vi "Generate Method Description.vi"(8 "error in (no error)":errorcluster, 10 "Test Method Result In":T1, 11 "Test Tree In":refnum<class "Test Result Tree.lvclass">) -> (0 "error out":errorcluster, 3 "Test Tree Out":refnum<class "Test Result Tree.lvclass">)   [LabVIEW 2020, in "Test Result Tree.lvclass"]
uses:
  Test Result Tree/Test Result Tree.lvclass
  Result Types/Method Result/Method Result.ctl
  Rewrite Project/Result/Status.ctl
  Result Types/Assertion Result/Assertion Result.ctl
  Result Types/Assertion Result/Public/TypeDefs/Assertion Type.ctl
  C:/Git/astemes-lunit/source/Framework/Helper Classes/Test Tree/Test Tree.lvclass
  Test Tree.lvclass/Test Tree.ctl
  Test Tree.lvclass
  Result Types/Assertion Result/Assertion Result.lvlib
  Result Types/Method Result/Method Result.lvlib
  Rewrite Project/Result/Result.lvlib
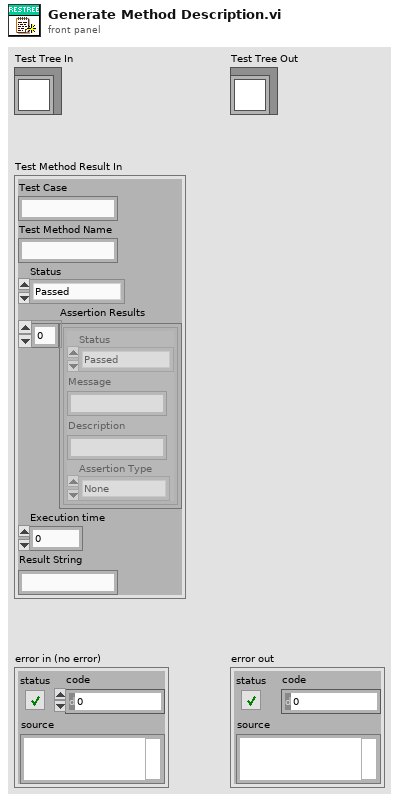
[diagram p1: front panel]
types:
  T1 = typedef "Method Result.lvlib/Method Result.ctl" = cluster{"Test Case":string, "Test Method Name":string, "Status":T2, "Assertion Results":T3[], "Execution time":dbl, "Result String":string}
  T2 = typedef "Result.lvlib/Status.ctl" = enum16{"Passed", "Failed", "Error", "Skipped", "Setup Error", "Broken", "Teardown Error"}
  T3 = typedef "Assertion Result.lvlib/Assertion Result.ctl" = cluster{"Status":T2, "Message":string, "Description":string, "Assertion Type":T4}
  T4 = typedef "Result.lvlib/Assertion Type.ctl" = enum16{"None", "Pass", "Fail", "Skip", "Pass if Equal", "Fail if Equal", "Pass if Error", "Fail if Error", "Pass if", "Fail if"}
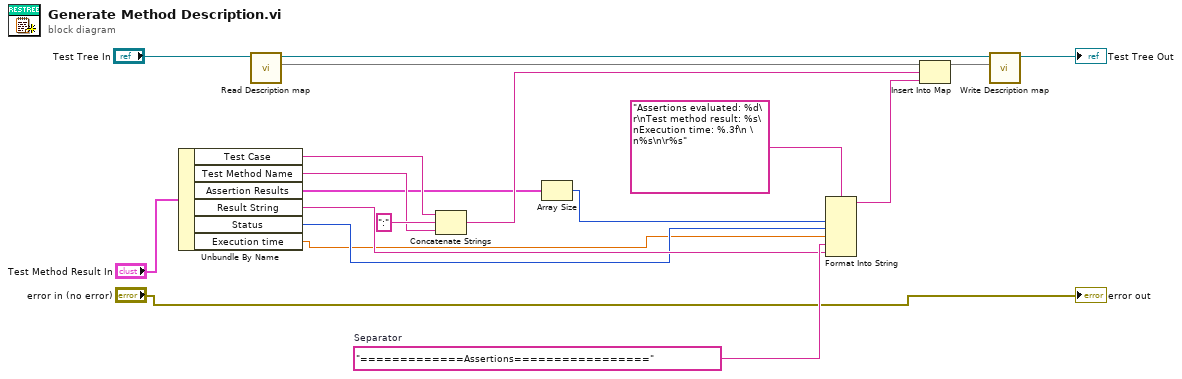
[diagram p0: block diagram]
diagram:
  w15 = "=============Assertions================="  # Separator
  n1 = Unbundle By Name("Test Method Result In") -> ("Test Case"=w7:string, "Test Method Name"=w6:string, "Assertion Results"=w5:T3[], "Result String"=w3:string, "Status"=w2:T2, "Execution time"=w1:dbl)
  n2 = call "Read Description map.vi"("Test Tree in"="Test Tree In") -> ("Description map"=w10:map{string, string}, "Test Tree out"=w11:refnum<class "Test Result Tree.lvclass">)  [unwired: 8 in, 1 out]
  n3 = Concatenate Strings(w7, ":" ("string"), w6) -> (w19:string)
  n4 = Array Size(array=w5) -> (size(s)=w4:i32)
  n5 = Format Into String(format string="Assertions evaluated: %d\r\nTest method result: %s\nExecution time: %.3f\n \n%s\n\r%s", w4, w2, w1, w15, w3) -> (resulting string=w16:string)  [unwired: 2 in, 1 out]
  n6 = Insert Into Map(map in=w10, key=w19, value=w16) -> (map out=w13:map{string, string})  [unwired: 2 out]
  n7 = call "Write Description map.vi"("Description map"=w13, "Test Tree in"=w11) -> ("Test Tree out"=→"Test Tree Out":refnum<class "Test Result Tree.lvclass">)  [unwired: 8 in, 1 out]
  "error out" <- "error in (no error)"
